vi "replaceAutoManDialog.vi"() -> (3 "T button?":bool)   [LabVIEW 2014]
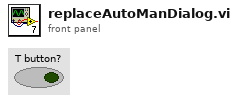
[diagram p1: front panel]
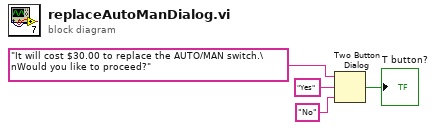
[diagram p0: block diagram]
diagram:
  n1 = Two Button Dialog(message="It will cost $30.00 to replace the AUTO/MAN switch.\nWould you like to proceed?", 1:"No" ("F button name (\"Cancel\")"), 2:"Yes" ("T button name (\"OK\")")) -> (T button?=→"T button?":bool)
